vi "Rename setget methods and set icon.vi"() -> ()   [LabVIEW 2012]
uses:
  <vilib>/LabVIEW Icon API/API_User Layer Data.ctl
  <vilib>/Utility/miscctls.llb/LVPoint32TypeDef.ctl
  <vilib>/picture/picture.llb/imagedata.ctl
  <vilib>/LabVIEW Icon API/LabVIEW Icon API.lvlib
panel:
  in  "My Computer?":bool
  in  "Project Path":path
  in  "Folder Path":path
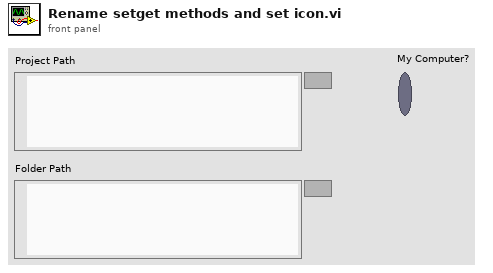
[diagram p1: front panel]
types:
  T1 = typedef "LVPoint32TypeDef.ctl" = cluster{"Horizontal":i32, "Vertical":i32}
  T2 = typedef "LabVIEW Icon API.lvlib/API_User Layer Data.ctl" = cluster{"Layer name":string, "Origin":T1, "Icon image data":T3}
  T3 = typedef "imagedata.ctl" = cluster{"image type":i32, "image depth":i32, "image":u8[], "mask":u8[], "colors":u32[], "Rectangle":cluster{"left":i16, "top":i16, "right":i16, "bottom":i16}}
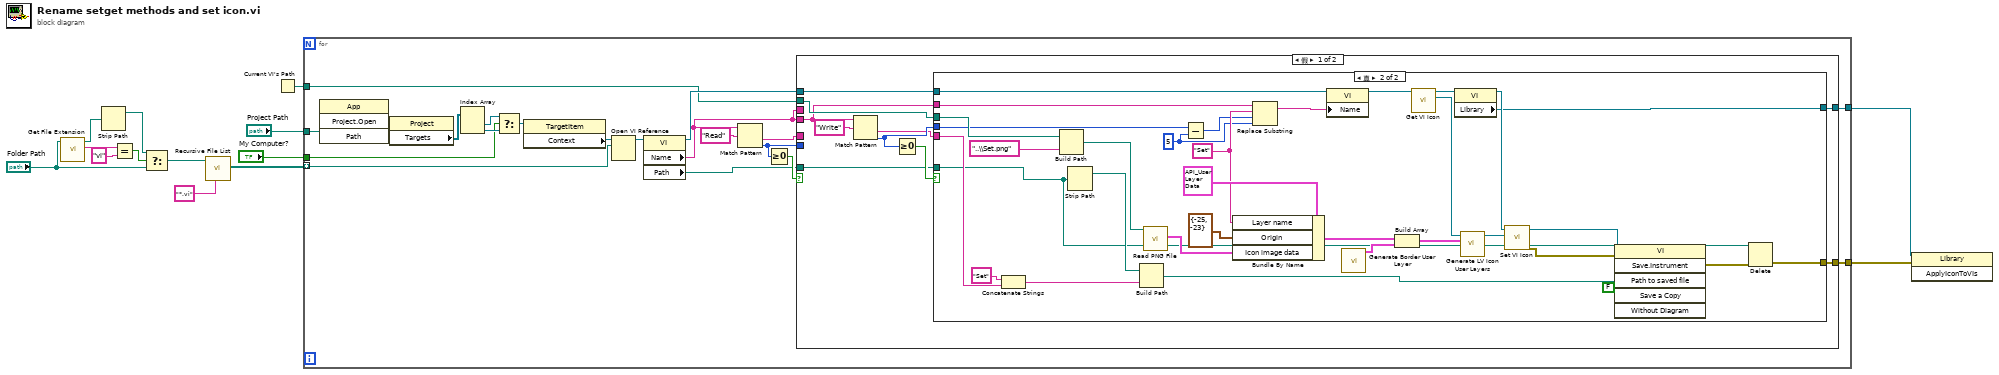
[diagram p0: block diagram]
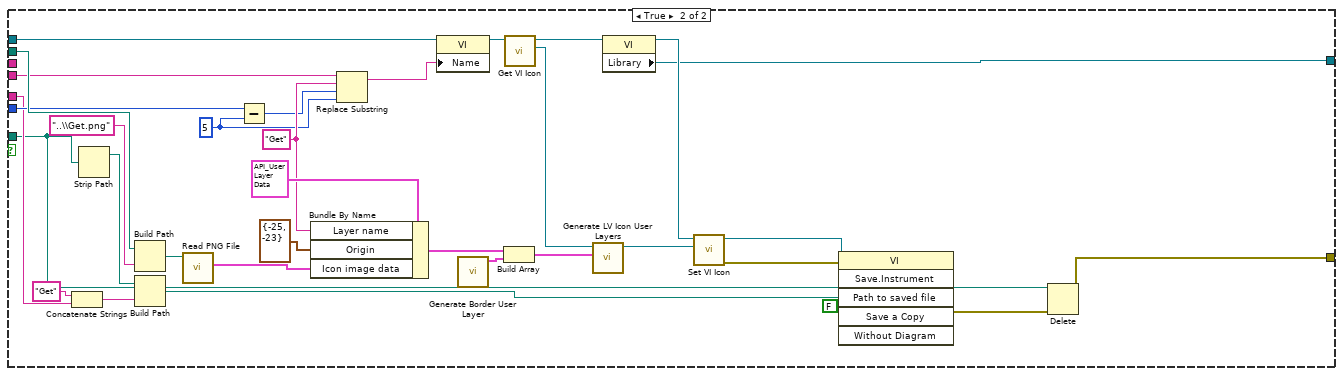
[diagram p3: hidden frame]
diagram:
  n1 = call <vilib>:"Get File Extension.vi"("file"="Folder Path") -> ("lowercase file extension"=w9:string, "dup file"=w6:path)  [unwired: 7 in, 2 out]
  n2 = Strip Path(path=w6) -> (stripped path=w5:path)  [unwired: 1 out]
  n3 = Equal?(x=w9, y="vi") -> (x = y?=w7:bool)
  n4 = Select(t=w5, s=w7, f="Folder Path") -> (s? t:f=w4:path)
  n5 = call <vilib>:"Recursive File List.vi"("pattern"="*.vi", "Folder Path"=w4) -> ("All Files in Dir"=w13:path[])  [unwired: 5 in, 4 out]
  n6 = Current VI's Path() -> (path=w10:path)
  n7 = for {
    tunnel: w13 -> [w21] mode=indexing
    tunnel: "My Computer?" -> [w28]
    tunnel: "Project Path" -> [w27]
    tunnel: w10 -> [w22]
    tunnel: [w16] -> w2
    tunnel: [w15] -> w1
    n8 = invoke class="App" method="Project.Open"("Path"=w27) -> ("Project:Open"=w33:refnum<vi>)  [unwired: 3 in, 3 out]
    n9 = property class="Project"(reference=w33) -> ("Targets"=w32:refnum<vi>[])  [unwired: 1 in, 2 out]
    n10 = Index Array(array=w32) -> (element #1=w31:refnum<vi>, element #2=w30:refnum<vi>)  [unwired: 2 in]
    n11 = Select(t=w31, s=w28, f=w30) -> (s? t:f=w29:refnum<vi>)
    n12 = property class="TargetItem"(reference=w29) -> ("Context"=w34:refnum<vi>)  [unwired: 1 in, 2 out]
    n13 = Open VI Reference(application reference (local)=w34, vi path=w21) -> (vi reference=w26:refnum<vi>)  [unwired: 4 in, 1 out]
    n14 = property class="VI"(reference=w26) -> (reference out=w23:refnum<vi>, "Name"=w20:string, "Path"=w18:path)  [unwired: 1 in, 1 out]
    n15 = Match Pattern(string=w20, regular expression="Read") -> (after substring=w17:string, offset past match=w19:i32)  [unwired: 1 in, 2 out]
    n16 = Greater Or Equal To 0?(x=w19) -> (x >= 0?=w24:bool)
    n17 = case shown="假" w24 {
      tunnel: w23 -> [w42 w110]
      tunnel: w22 -> [w41 w109]
      tunnel: w20 -> [w40 w108]
      tunnel: w20 -> [_ _]
      tunnel: w19 -> [_ w89]
      tunnel: w18 -> [w38 w81]
      tunnel: w17 -> [_ w87]
      tunnel: [w36 w80] -> w16
      tunnel: [w35 w79] -> w15
      frame False {
        n18 = Match Pattern(string=w40, regular expression="Write") -> (after substring=w37:string, offset past match=w39:i32)  [unwired: 1 in, 2 out]
        n19 = Greater Or Equal To 0?(x=w39) -> (x >= 0?=w43:bool)
        n20 = case shown="真" w43 {
          tunnel: w42 -> [_ w67]
          tunnel: w41 -> [_ w66]
          tunnel: w40 -> [_ w64]
          tunnel: w39 -> [_ w61]
          tunnel: w38 -> [_ w48]
          tunnel: w37 -> [_ w52]
          tunnel: [_ w47] -> w36
          tunnel: [_ w45] -> w35
          frame False {
          }
          frame True {
            w59 = 5 ("length (len. of substring)")
            w65 = "Set"
            n21 = Concatenate Strings("Set" ("string"), w52) -> (w54:string)
            n22 = Build Path(base path=w66, name or relative path="..\\Set.png") -> (appended path=w73:path)
            n23 = Strip Path(path=w48) -> (stripped path=w55:path)  [unwired: 1 out]
            n24 = Build Path(base path=w55, name or relative path=w54) -> (appended path=w51:path)
            n25 = call <vilib>:"Read PNG File.vi"("path to PNG file"=w73) -> ("image data"=w72:T3)  [unwired: 8 in, 2 out]
            n26 = Subtract(x=w61, y=w59) -> (x-y=w60:i32)
            n27 = Bundle By Name(cluster=T2 {"Layer name"="", "Origin"={"Horizontal"=0, "Vertical"=0}, "Icon image data"={"image type"=0, "image depth"=0, "image"=[], "mask"=[], "colors"=[], "Rectangle"={"left"=0, "top"=0, "right"=0, "bottom"=0}}} ("User layer"), "Layer name"=w65, "Origin"=T1 {"Horizontal"=-25, "Vertical"=-23}, "Icon image data"=w72) -> (w70:T2)
            n28 = Replace Substring(2:w59, 3:w60, 4:w65, 5:w64) -> (1:w63:string)  [unwired: 1 out]
            n29 = property class="VI"(reference=w67, "Name"=w63) -> (reference out=w77:refnum<vi>)  [unwired: 1 in, 1 out]
            n30 = call <vilib>:"Generate Border User Layer.vi"() -> ("User Layer data"=w62:T2)  [unwired: 11 in]
            n31 = Build Array(w70, w62) -> (w69:T2[])
            n32 = call <vilib>:"Get VI Icon.vi"("VI Refnum in"=w77) -> ("Icon"=w76:refnum<class "Icon.lvclass">, "VI Refnum out"=w58:refnum<vi>)  [unwired: 8 in, 1 out]
            n33 = property class="VI"(reference=w58) -> (reference out=w57:refnum<vi>, "Library"=w45:refnum<vi>)  [unwired: 1 in, 1 out]
            n34 = call <vilib>:"Generate LV Icon User Layers.vi"("User layers"=w69, "Icon in"=w76) -> ("Icon out"=w56:refnum<class "Icon.lvclass">)  [unwired: 8 in, 1 out]
            n35 = call <vilib>:"Set VI Icon.vi"("Icon"=w56, "VI Refnum in"=w57) -> ("error out"=w46:errorcluster, "VI Refnum out"=w68:refnum<vi>)  [unwired: 8 in]
            n36 = invoke class="VI" method="Save.Instrument"(reference=w68, error in=w46, "Path to saved file"=w51, "Save a Copy"=FALSE) -> (error out=w49:errorcluster)  [unwired: 2 in, 5 out]
            n37 = Delete(path (use dialog)=w48, error in=w49) -> (error out=w47:errorcluster)  [unwired: 3 in, 2 out]
          }
        }
      }
      frame True {
        w93 = 5 ("length (len. of substring)")
        w97 = "Get"
        n38 = Concatenate Strings("Get" ("string"), w87) -> (w86:string)
        n39 = Strip Path(path=w81) -> (stripped path=w88:path)  [unwired: 1 out]
        n40 = Build Path(base path=w109, name or relative path="..\\Get.png") -> (appended path=w103:path)
        n41 = Build Path(base path=w88, name or relative path=w86) -> (appended path=w84:path)
        n42 = call <vilib>:"Read PNG File.vi"("path to PNG file"=w103) -> ("image data"=w102:T3)  [unwired: 8 in, 2 out]
        n43 = Subtract(x=w89, y=w93) -> (x-y=w94:i32)
        n44 = Bundle By Name(cluster=T2 {"Layer name"="", "Origin"={"Horizontal"=0, "Vertical"=0}, "Icon image data"={"image type"=0, "image depth"=0, "image"=[], "mask"=[], "colors"=[], "Rectangle"={"left"=0, "top"=0, "right"=0, "bottom"=0}}} ("User layer"), "Layer name"=w97, "Origin"=T1 {"Horizontal"=-25, "Vertical"=-23}, "Icon image data"=w102) -> (w100:T2)
        n45 = Replace Substring(2:w93, 3:w94, 4:w97, 5:w108) -> (1:w96:string)  [unwired: 1 out]
        n46 = property class="VI"(reference=w110, "Name"=w96) -> (reference out=w107:refnum<vi>)  [unwired: 1 in, 1 out]
        n47 = call <vilib>:"Generate Border User Layer.vi"() -> ("User Layer data"=w95:T2)  [unwired: 11 in]
        n48 = Build Array(w100, w95) -> (w99:T2[])
        n49 = call <vilib>:"Get VI Icon.vi"("VI Refnum in"=w107) -> ("Icon"=w106:refnum<class "Icon.lvclass">, "VI Refnum out"=w92:refnum<vi>)  [unwired: 8 in, 1 out]
        n50 = call <vilib>:"Generate LV Icon User Layers.vi"("User layers"=w99, "Icon in"=w106) -> ("Icon out"=w90:refnum<class "Icon.lvclass">)  [unwired: 8 in, 1 out]
        n51 = property class="VI"(reference=w92) -> (reference out=w91:refnum<vi>, "Library"=w79:refnum<vi>)  [unwired: 1 in, 1 out]
        n52 = call <vilib>:"Set VI Icon.vi"("Icon"=w90, "VI Refnum in"=w91) -> ("error out"=w78:errorcluster, "VI Refnum out"=w98:refnum<vi>)  [unwired: 8 in]
        n53 = invoke class="VI" method="Save.Instrument"(reference=w98, error in=w78, "Path to saved file"=w84, "Save a Copy"=FALSE) -> (error out=w82:errorcluster)  [unwired: 2 in, 5 out]
        n54 = Delete(path (use dialog)=w81, error in=w82) -> (error out=w80:errorcluster)  [unwired: 3 in, 2 out]
      }
    }
  }
  n55 = invoke class="Library" method="ApplyIconToVIs"(reference=w1, error in=w2) -> ()  [unwired: 1 in, 3 out]
